vi "SFID datastream - external control.vi"(3 "Data rate set (Hz)":dbl=100.0, 4 "N samples":u32=1000, 5 "COM port":refnum<visa-resource-name>) -> (0 "Error out":errorcluster, 1 "Data rate returned (Hz)":dbl=100.0, 2 "Data cluster array out":T1[](array[typedef]))   [LabVIEW 2022 SP3]
uses:
  Ctls/SFID_Data.ctl
  Ctls/SFID_Cmd.ctl
panel:
  out "Environment chart":T2(graph)
  in  "Stop Button":bool
  out "Voltage chart":sgl(graph)
  # "Vout (V)"
  # "P0 (Pa)"
  # "T (°C)"
  # "RH (%)"
  # "Surrey Sensors 08/2024  v1.0"
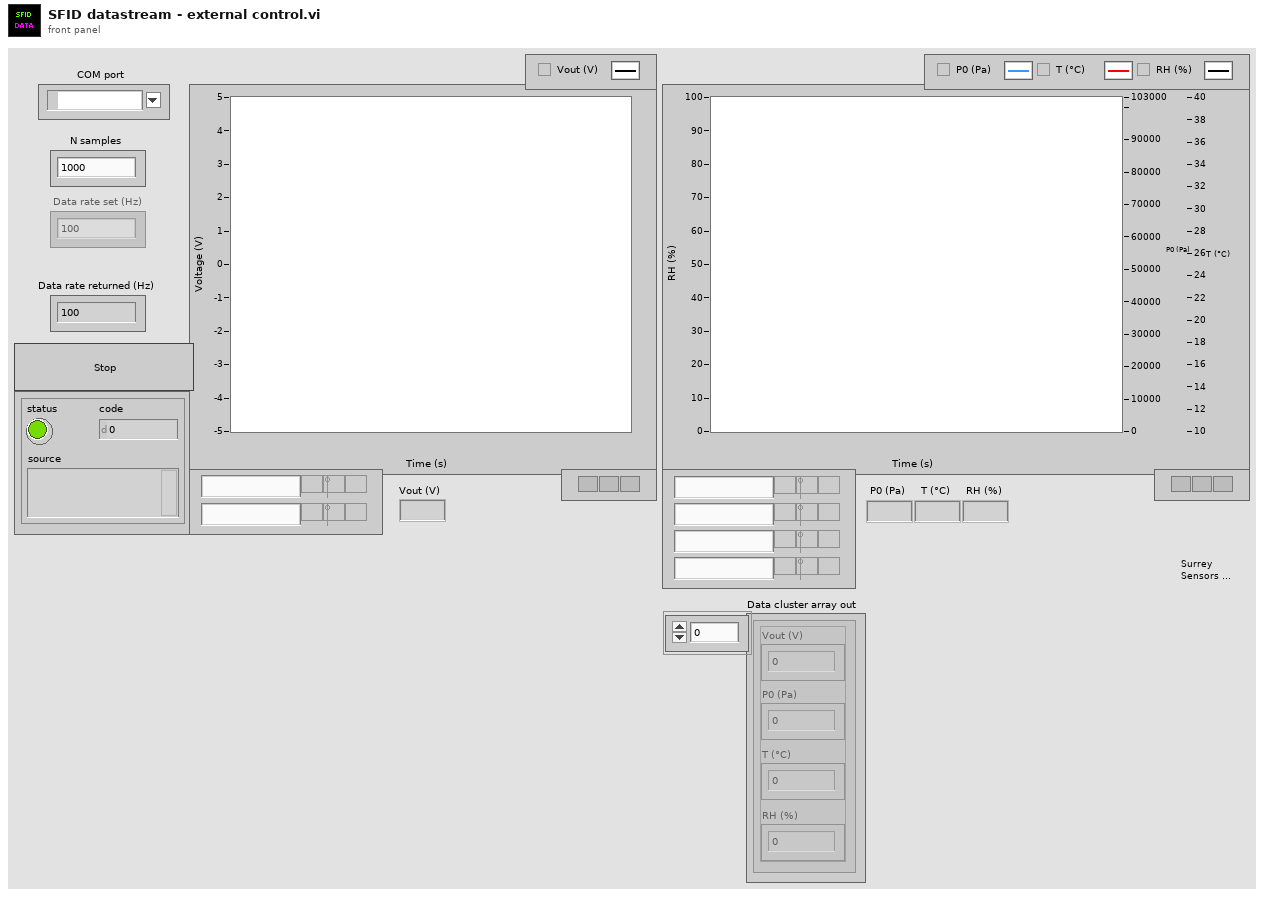
[diagram p1: front panel]
types:
  T1 = typedef "SFID_Data.ctl" = cluster{"Vout (V)":sgl, "P0 (Pa)":sgl, "T (°C)":sgl, "RH (%)":sgl}
  T2 = cluster{"P0 (Pa)":sgl, "T (°C)":sgl, "RH (%)":sgl}
  T3 = cluster{"P0 (Pa)":sgl, "T (°C)":sgl, "RH (%)":sgl}[]
  T4 = typedef "SFID_Cmd.ctl" = string
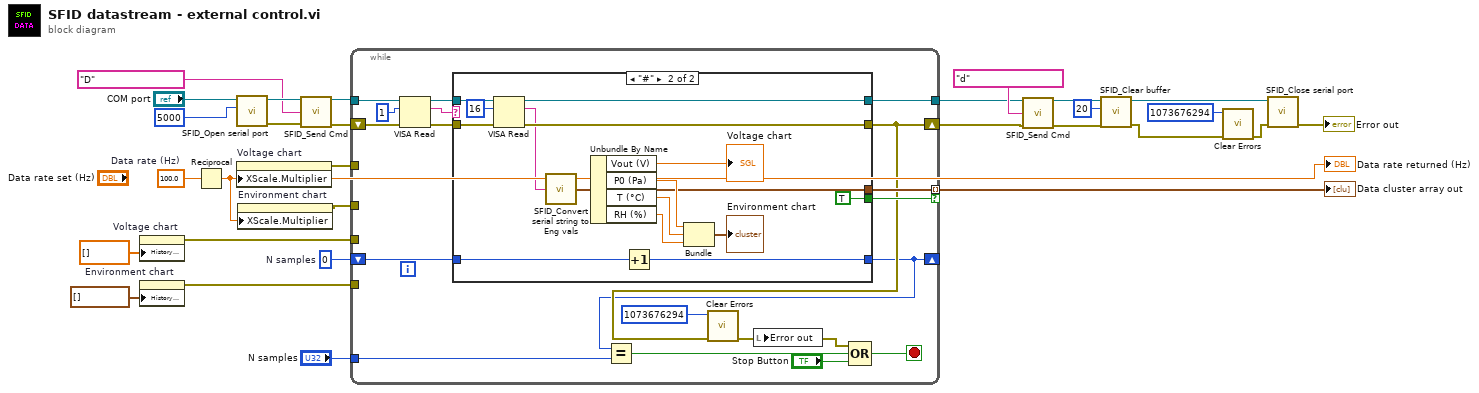
[diagram p0: block diagram]
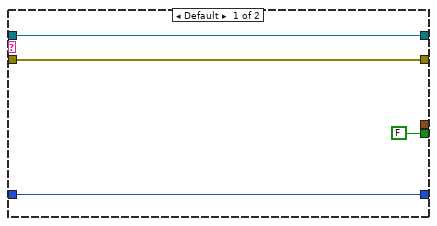
[diagram p2: hidden frame]
diagram:
  w10 = u32 0  # N samples
  w1 = 100.0  # Data rate (Hz)
  n1 = property on="Voltage chart" class="WFChart (strict)"("History Data"=sgl[] []) -> (error out=w5:errorcluster)  [unwired: 2 in, 1 out]
  n2 = property on="Environment chart" class="WFChart (strict)"("History Data"=T3 []) -> (error out=w2:errorcluster)  [unwired: 2 in, 1 out]
  n3 = Reciprocal(x=w1) -> (1/x=w7:dbl)
  n4 = call "SFID_Open serial port.vi"("timeout (ms)"=u32 5000, "VISA resource name"="COM port") -> ("Error out"=w19:errorcluster, "VISA resource name out"=w21:refnum<visa-resource-name>)  [unwired: 8 in]
  n5 = property on="Voltage chart" class="WFChart (strict)"("XScale.Multiplier"=w7) -> (error out=w16:errorcluster)  [unwired: 2 in, 1 out]
  n6 = property on="Environment chart" class="WFChart (strict)"("XScale.Multiplier"=w7) -> (error out=w6:errorcluster)  [unwired: 2 in, 1 out]
  n7 = call "SFID_Send Cmd.vi"("Port"=w21, "Cmd"=T4 "D", "Error In"=w19) -> ("Port out"=w18:refnum<visa-resource-name>, "Error Out"=w17:errorcluster)  [unwired: 11 in]
  n8 = while {
    shift-right: [w36] -> w22
    shift-left: w17 -> [w41]
    tunnel: w16 -> [_]
    tunnel: w18 -> [w42]
    tunnel: [w43] -> w23
    shift-right: [w33] -> _
    shift-left: w10 -> [w40]
    tunnel: [w39] -> w8 mode=indexing if=w38
    tunnel: "N samples" -> [w34]
    tunnel: w6 -> [_]
    tunnel: w5 -> [_]
    tunnel: w2 -> [_]
    stop <- w32 stop-if-true
    n9 = VISA Read(VISA resource name=w42, byte count=u32 1, error in (no error)=w41) -> (VISA resource name out=w45:refnum<visa-resource-name>, read buffer=w46:string, error out=w44:errorcluster)  [unwired: 1 out]
    n10 = case shown="\"#\"" w46 {
      tunnel: w45 -> [w50 w66]
      tunnel: w44 -> [w51 w65]
      tunnel: [w50 w63] -> w43
      tunnel: [w51 w62] -> w36
      tunnel: w40 -> [w49 w60]
      tunnel: [w49 w59] -> w33
      tunnel: [_ w52] -> w39
      tunnel: [FALSE TRUE] -> w38
      frame Default {
      }
      frame "#" {
        n11 = VISA Read(VISA resource name=w66, byte count=u32 16, error in (no error)=w65) -> (VISA resource name out=w63:refnum<visa-resource-name>, read buffer=w61:string, error out=w62:errorcluster)  [unwired: 1 out]
        n12 = call "SFID_Convert serial string to Eng vals.vi"("Serial buffer string (excluding FrameChar)"=w61) -> ("SFID data"=w52:T1)
        n13 = Unbundle By Name(w52) -> ("Vout (V)"=→"Voltage chart":sgl, "P0 (Pa)"=w57:sgl, "T (°C)"=w56:sgl, "RH (%)"=w55:sgl)
        n14 = Increment(x=w60) -> (x+1=w59:u32)
        n15 = Bundle("P0 (Pa)"=w57, "T (°C)"=w56, "RH (%)"=w55) -> (→"Environment chart":T2)  [unwired: 1 in]
      }
    }
    n16 = Equal?(x=w33, y=w34) -> (x = y?=w31:bool)
    n17 = call <vilib>:"Clear Errors.vi"("error in (no error)"=w36, "specific error code to clear (0: all)"=1073676294) -> ("error out"=w35:errorcluster)  [unwired: 4 in, 1 out]
    n18 = local write "Error out"(w35) -> ()
    n19 = Compound Arithmetic op=OR(w35, w31, "Stop Button") -> (w32:bool)
  }
  "Data cluster array out" <- w8
  n20 = call "SFID_Send Cmd.vi"("Port"=w23, "Cmd"=T4 "d", "Error In"=w22) -> ("Port out"=w12:refnum<visa-resource-name>, "Error Out"=w11:errorcluster)  [unwired: 11 in]
  n21 = call "SFID_Clear buffer.vi"("Error in"=w11, "dt for timeout (ms)"=u32 20, "VISA resource name in"=w12) -> ("Error out"=w13:errorcluster, "VISA resource name out"=w14:refnum<visa-resource-name>)  [unwired: 3 in]
  n22 = call <vilib>:"Clear Errors.vi"("error in (no error)"=w13, "specific error code to clear (0: all)"=1073676294) -> ("error out"=w26:errorcluster)  [unwired: 4 in, 1 out]
  n23 = call "SFID_Close serial port.vi"("Error in"=w26, "VISA resource name"=w14) -> ("Error out"=→"Error out":errorcluster)  [unwired: 9 in]
  "Data rate returned (Hz)" <- w1
